vi "CANopen Read TPDO.vi"() -> ()   [LabVIEW 2016]
doc: "This example demonstrates how to read CANopen TPDO data from the device."
uses:
  <vilib>/userdefined/High Color/nirio_resource_hc.ctl
  <vilib>/Platform/TimedLoop/XDataNode/timing_clust.ctl
  <vilib>/Platform/TimedLoop/XDataNode/nitl_modes.ctl
  <vilib>/Platform/TimedLoop/XDataNode/wakeup.ctl
  <vilib>/FPGAPlugInAG/cRIO-9033/niLvFpga_Open_cRIO-9033.vi
  <vilib>/rvi/interface/common/dynamic/niFpgaDynamicAddResources.vi
  <vilib>/CANopenLib/CANOPEN.llb/CANopen Interface Create.vi
  <vilib>/CANopenLib/CANOPEN.llb/CANopen TPDO Create.vi
  <vilib>/CANopenLib/CANOPEN.llb/CANopen TPDO Start.vi
  <vilib>/CANopenLib/CANOPEN.llb/CANopen Fetch from Data [U8].vi
  <vilib>/CANopenLib/CANOPEN.llb/CANopen TPDO Close.vi
  <vilib>/CANopenLib/CANOPEN.llb/CANopen Interface Close.vi
  <vilib>/FPGAPlugInAG/Dynamic/niLvFpga_Close_Dynamic.vi
  <vilib>/rvi/interface/nirviOpenFPGA/nirviOpenFPGA.xnode
  Users/s163601/Desktop/05-28/FPGA Bitfiles/project_FPGATarget_FPGAMain_kDJZXzfRsH0.lvbitx
  robotics/EPOS2 CANOpen Driver/FPGA/FPGA Main.vi
  <vilib>/Platform/TimedLoop/XDataNode/XDataNode.xnode
  <vilib>/rvi/interface/nirviCloseFPGA/nirviCloseFPGA.xnode
  <vilib>/Platform/TimedLoop/XDataNode/XDNodeRunTimeDep.lvlib
panel:
  in  "error in":errorcluster
  out "TPDO data":u8[](array[numeric])
  in  "buffer size (0)":u16=10
  in  "period (ms)":i64=10
  in  "stop":bool
  out "New data?":bool
  out "timestamp":timestamp
  in  "offset (0)":u32
  out "first value":u8
  in  "PDO channel":u8(ring) items=["PDO 1", "PDO 2", "PDO 3", "PDO 4"]
  in  "node-ID":u8=1 min=1 max=127 step=1
  in  "baud rate":u32(ring)=2 items=["1 Mbit/s"=0, "800 kbit/s"=1, "500 kbit/s"=2, "250 kbit/s"=3, "125 kbit/s"=4, "50 kbit/s"=6, "20 kbit/s"=7, "10 kbit/s"=8]
  in  "CANopen interface":u32(ring) items=["CANopen01", "CANopen02", "CANopen03", "CANopen04", "CANopen05", "CANopen06", "CANopen07", "CANopen08", "CANopen09", "CANopen10", "CANopen11", "CANopen12", "CANopen13", "CANopen14", "CANopen15", "CANopen16", "CANopen17", "CANopen18", "CANopen19", "CANopen20", "CANopen21", "CANopen22", "CANopen23", "CANopen24", "CANopen25", "CANopen26", "CANopen27", "CANopen28", "CANopen29", "CANopen30", "CANopen31", "CANopen32"]
  # "Overview: This example demonstrates how to read CANopen TPDO data from the device.\nRequirements: Connect CANopen module with a slave device. \nInstructions:\n1. Specify the values of CANopen interface, baud rate of the CANopen interface, node-ID of the slave device and \n    buffer size (0) of the maximum number of CAN frames that the TPDO receive buffer saves.\n2. Run this VI.\n3. Click STOP to stop the VI."
  # "Create CANopen interface and RPDO object"
  # "Read TPDO data"
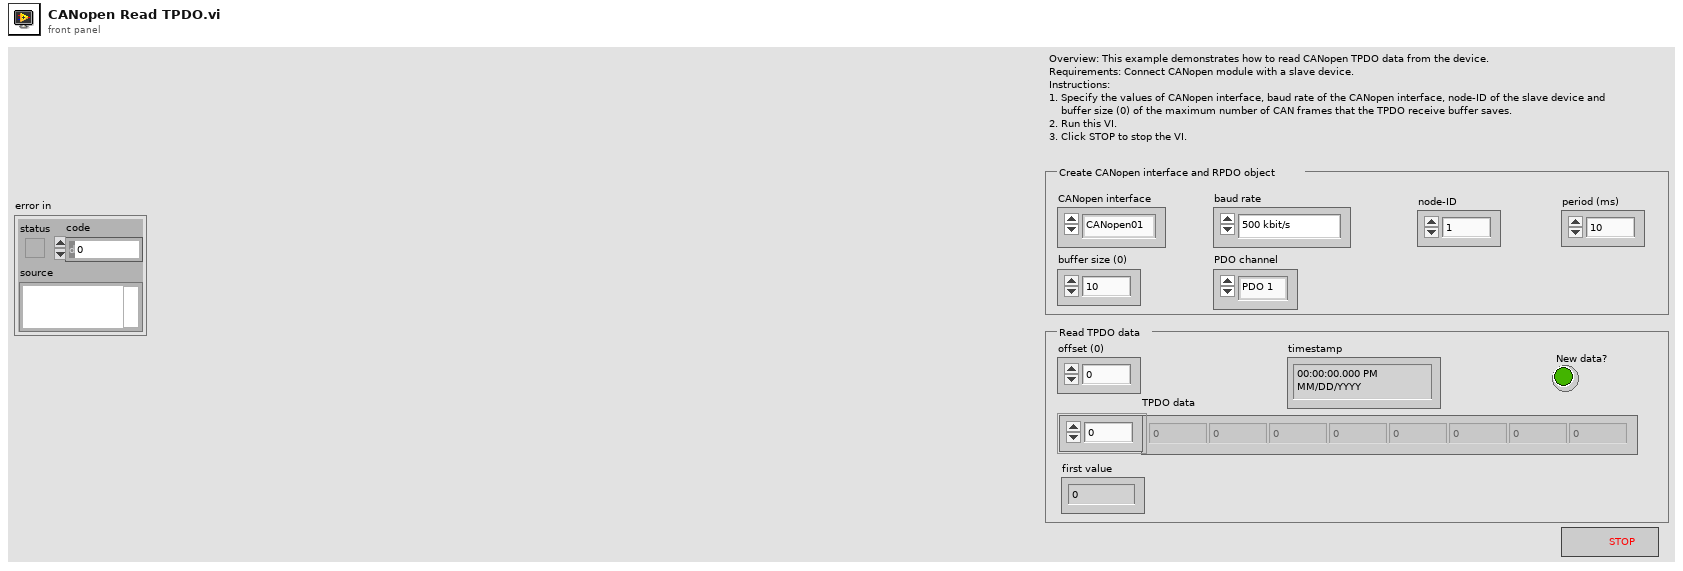
[diagram p1: front panel]
types:
  T1 = typedef "nirio_resource_hc.ctl" = tag
  T2 = typedef "XDNodeRunTimeDep.lvlib/timing_clust.ctl" = cluster{"Expected End [f-1]":u64, "Actual End [f-1]":u64, "Finished Late? [f-1]":bool, "Expected End [i-1]":u64, "Actual End [i-1]":u64, "Finished Late? [i-1]":bool, "Expected Start [i]":u64, "Actual Start [i]":u64, "Expected Start [f]":u64, "Actual Start [f]":u64, "Source Name":string, "Structure Name":string, "Period":i64, "Deadline":i64, "Offset":i64, "Start":i64, "Priority":i32, "Timeout":i32, "Mode":T3, "Wakeup Reason":T4, "Error":errorcluster, "Source Type":string, "Secondary Source Type":string, "Global End Time":u64, "Global Start Time":u64, "Frame Duration":u64, "Iteration Duration":u64, "Assigned CPU":i32, "I/O Scan Engine Mode":u32}
  T3 = typedef "XDNodeRunTimeDep.lvlib/nitl_modes.ctl" = enum32{"No Change", "Process missed periods, maintain original phase", "Discard missed periods, maintain original phase", "Process missed periods, ignore original phase", "Discard missed periods, ignore original phase"}
  T4 = typedef "XDNodeRunTimeDep.lvlib/wakeup.ctl" = enum32{"Normal", "Aborted", "Asynchronous wakeup", "Timing source error", "Timed loop error", "Timeout"}
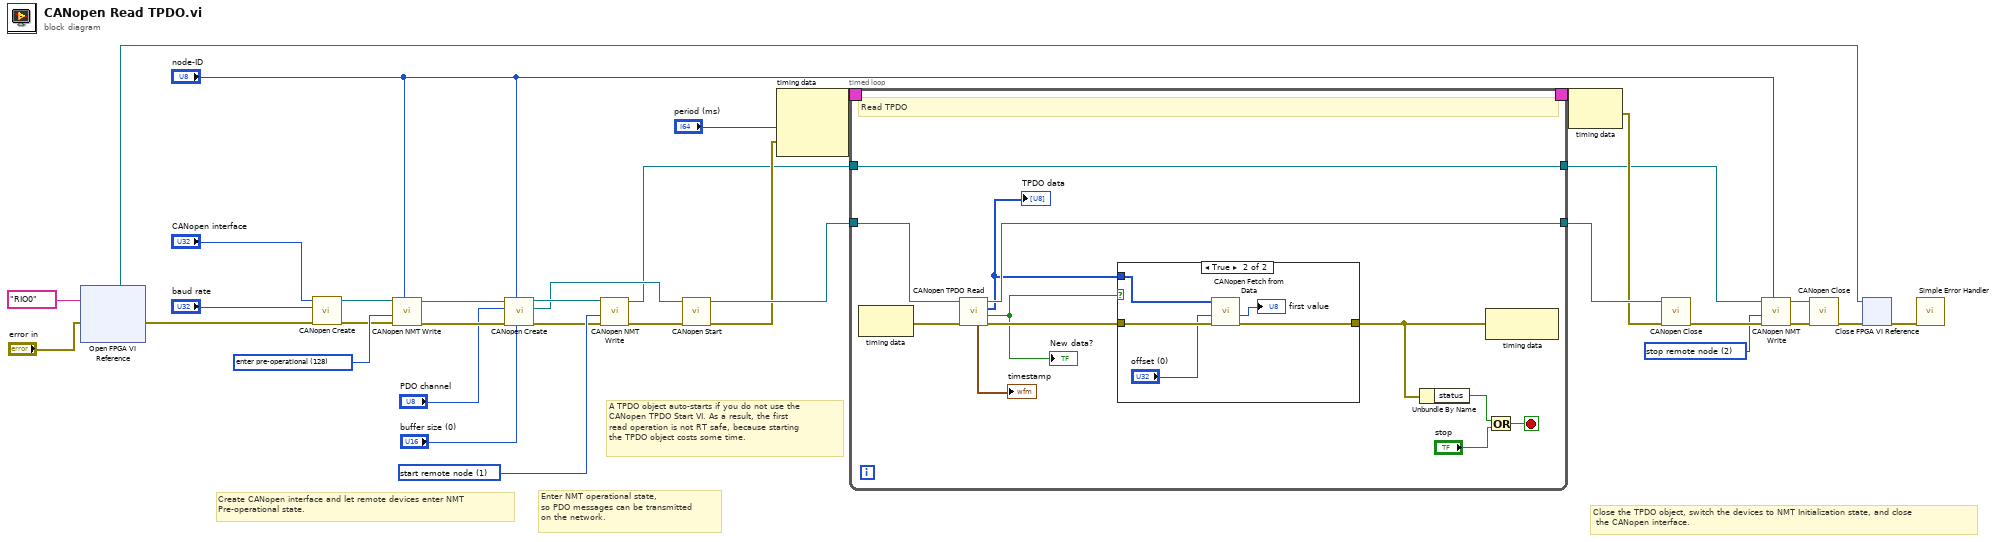
[diagram p0: block diagram]
diagram:
  w16 = u16 1 items=["start remote node"=1, "stop remote node"=2, "enter pre-operational"=128, "reset node"=129, "reset communication"=130] ("command")
  w20 = u16 2 items=["start remote node"=1, "stop remote node"=2, "enter pre-operational"=128, "reset node"=129, "reset communication"=130] ("command")
  w28 = u16 128 items=["start remote node"=1, "stop remote node"=2, "enter pre-operational"=128, "reset node"=129, "reset communication"=130] ("command")
  # "A TPDO object auto-starts if you do not use the \nCANopen TPDO Start VI. As a result, the first \nread operation is not RT safe, because starting \nthe TPDO object costs some time."
  # "Close the TPDO object, switch the devices to NMT Initialization state, and close\n the CANopen interface."
  # "Create CANopen interface and let remote devices enter NMT\nPre-operational state."
  # "Enter NMT operational state,\nso PDO messages can be transmitted\non the network."
  n1 = xnode ("Open FPGA VI Reference")("error in"="error in", "resource name"=T1 "RIO0") -> ("FPGA VI Reference Out"=w1:refnum<k20>, "error out"=w4:errorcluster)
  n2 = call-poly <vilib>:"CANopen Create.vi"("error in (no error)"=w4, "baud rate"="baud rate", "interface name"="CANopen interface") -> ("error out"=w10:errorcluster, "interface object out"=w27:refnum<k20>)  [unwired: 7 in]
  n3 = call <vilib>:"CANopen NMT Write.vi"("node-ID (0)"="node-ID", "error in (no error)"=w10, "command"=w28, "interface object in"=w27) -> ("error out"=w31:errorcluster, "interface object out"=w32:refnum<k20>)  [unwired: 6 in]
  n4 = call-poly <vilib>:"CANopen Create.vi"("buffer size (0)"="buffer size (0)", "node-ID"="node-ID", "error in (no error)"=w31, "PDO channel"="PDO channel", "interface object in"=w32) -> ("error out"=w14:errorcluster, "TPDO object out"=w13:refnum<k20>, "interface object out"=w17:refnum<k20>)  [unwired: 4 in]
  n5 = call <vilib>:"CANopen NMT Write.vi"("error in (no error)"=w14, "command"=w16, "interface object in"=w17) -> ("error out"=w15:errorcluster, "interface object out"=w9:refnum<k20>)  [unwired: 7 in]
  n6 = call-poly <vilib>:"CANopen Start.vi"("error in (no error)"=w15, "TPDO object in"=w13) -> ("error out"=w12:errorcluster, "TPDO object out"=w24:refnum<k20>)  [unwired: 8 in]
  n7 = node-c288("period (ms)", w12) -> (w34:T2)  [unwired: 1 in]
  n8 = timed-loop {
    tunnel: [w43] -> w26
    tunnel: w24 -> [w46]
    timing: w34 -> [_]
    timing-out: [_] -> w33
    tunnel: w9 -> [w36]
    tunnel: [w36] -> w8
    stop <- w41 stop-if-true
    # "Read TPDO"
    n9 = node-c288() -> (w39:errorcluster)  [unwired: 1 in]
    n10 = call <vilib>:"CANopen TPDO Read.vi"("error in (no error)"=w39, "TPDO object in"=w46) -> ("error out"=w44:errorcluster, "new data?"=w40:bool, "data"=w37:u8[], "TPDO object out"=w43:refnum<k20>, "timestamp"=→"timestamp":timestamp)  [unwired: 5 in]
    "New data?" <- w40
    "TPDO data" <- w37
    n11 = case shown="True" w40 {
      tunnel: w44 -> [w52 w57]
      tunnel: w37 -> [_ w56]
      tunnel: [w52 w53] -> w35
      frame False {
      }
      frame True {
        n12 = call-poly <vilib>:"CANopen Fetch from Data.vi"("error in (no error)"=w57, "offset (0)"="offset (0)", "CANopen data in"=w56) -> ("error out"=w53:errorcluster, "unsigned 8-bit integer"=→"first value":u8)  [unwired: 6 in, 1 out]
      }
    }
    n13 = Unbundle By Name(w35) -> ("status"=w38:bool)
    n14 = node-c288(w35) -> ()  [unwired: 1 out]
    n15 = Or(x=w38, y="stop") -> (x .or. y?=w41:bool)
  }
  n16 = node-c288(w33) -> (w11:errorcluster)
  n17 = call-poly <vilib>:"CANopen Close.vi"("error in (no error)"=w11, "TPDO object in"=w26) -> ("error out"=w21:errorcluster)  [unwired: 9 in]
  n18 = call <vilib>:"CANopen NMT Write.vi"("node-ID (0)"="node-ID", "error in (no error)"=w21, "command"=w20, "interface object in"=w8) -> ("error out"=w23:errorcluster, "interface object out"=w22:refnum<k20>)  [unwired: 6 in]
  n19 = call-poly <vilib>:"CANopen Close.vi"("error in (no error)"=w23, "interface object in"=w22) -> ("error out"=w3:errorcluster)  [unwired: 9 in]
  n20 = xnode "Close FPGA VI Reference"("FPGA VI Reference In"=w1, "error in"=w3) -> ("error out"=w2:errorcluster)
  n21 = call <vilib>:"Simple Error Handler.vi"("error in (no error)"=w2) -> ()  [unwired: 4 in, 5 out]
